vi "Watts Up Series Real Time Graph.vi"() -> ()   [LabVIEW 2013]
doc: "Graph data from the Watts Up in a live-stream type format. This requires the use of <b>External logging mode</b> for the Watts Up device. The data will not be saved on the Watts Up meter but rather into the chart itself. To retrieve the data from the chart, right click and use <b>Export</b>.\n\nWhen <b>STOP</b> is pressed, the meter will be set back into internal logging mode (however the data will be cleared anytime the logging mode is changed)."
uses:
  <instrlib>/Watts Up Series/Watts Up Series.lvlib
panel:
  in  "Relay (ON)":bool=TRUE
  in  "Items To Graph":bool[](array[boolean])=[FALSE, FALSE, FALSE, FALSE, FALSE, FALSE, FALSE, FALSE, FALSE, FALSE, FALSE, FALSE, FALSE, FALSE, FALSE, FALSE, FALSE, FALSE]
  in  "Interval (10 s)":i32=10
  in  "?":bool
  out "Waveform Chart":T1(graph)
  in  "VISA resource name":refnum<visa-resource-name>
  # "(c) 2014 NATIONAL INSTRUMENTS.  ALL RIGHTS RESERVED."
  # "Watts"
  # "Volts"
  # "Amps"
  # "Watt Hours"
  # "Cost"
  # "WH/Month"
  # "Cost/Month"
  # "Wmax"
  # "Vmax"
  # "Amax"
  # "Wmin"
  # "Vmin"
  # "Amin"
  # "Power Factor"
  # "Duty Cycle"
  # "Power Cycle"
  # "Line Freq."
  # "Volt-Amps"
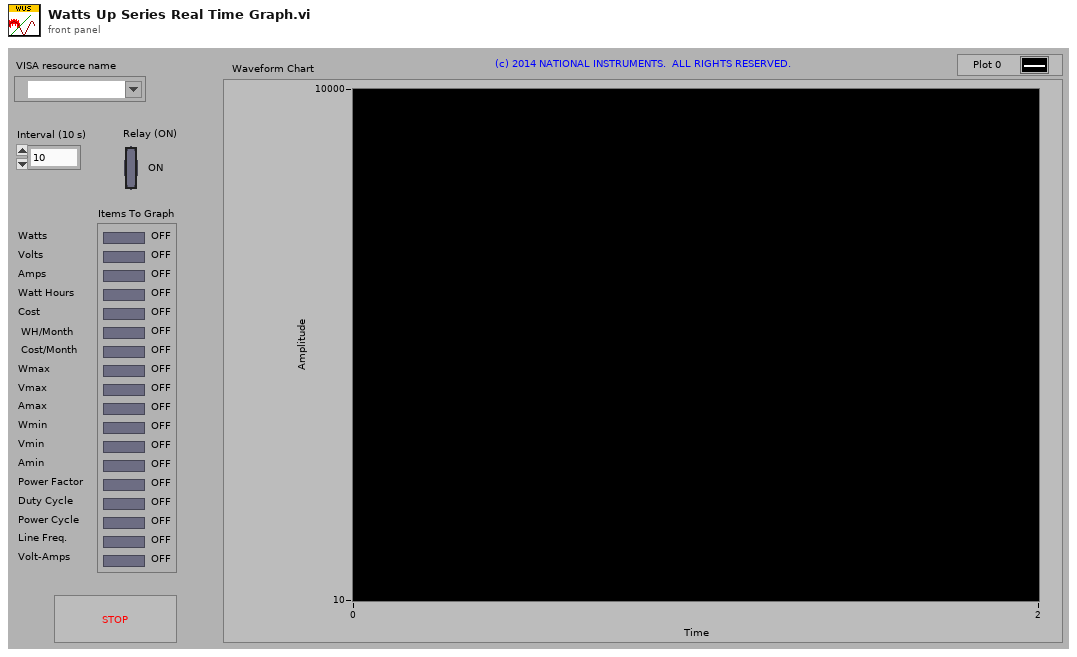
[diagram p1: front panel]
types:
  T1 = cluster{"Record[0]":dbl, "Record[1]":dbl, "Record[2]":dbl, "Record[3]":dbl, "Record[4]":dbl, "Record[5]":dbl, "Record[6]":dbl, "Record[7]":dbl, "Record[8]":dbl}
  T2 = cluster{"[0]":dbl, "[1]":dbl, "[2]":dbl, "[3]":dbl, "[4]":dbl, "[5]":dbl, "[6]":dbl, "[7]":dbl, "[8]":dbl}
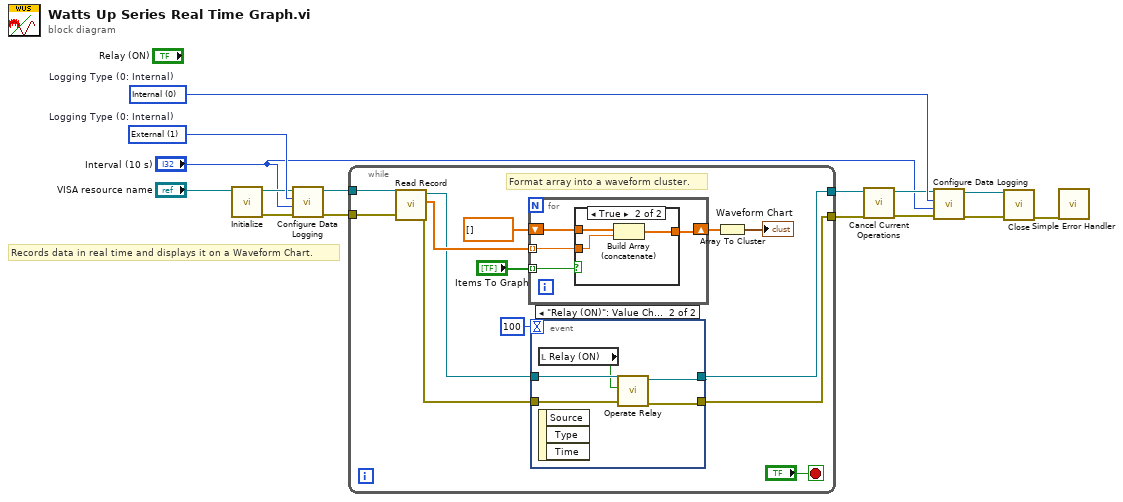
[diagram p0: block diagram]
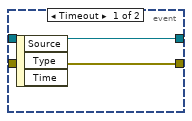
[diagram p2: hidden frame]
diagram:
  w10 = 0 items=["Internal", "External", "TCP"]  # Logging Type (0: Internal)
  w14 = 1 items=["Internal", "External", "TCP"]  # Logging Type (0: Internal)
  # "Records data in real time and displays it on a Waveform Chart."
  n1 = call <instrlib>:"Initialize.vi"("VISA resource name"="VISA resource name") -> ("error out"=w11:errorcluster, "VISA resource name out"=w12:refnum<visa-resource-name>)  [unwired: 9 in]
  n2 = call <instrlib>:"Configure Data Logging.vi"("error in (no error)"=w11, "Interval (10 s)"="Interval (10 s)", "Logging Type (0: Internal)"=w14, "VISA resource name"=w12) -> ("error out"=w2:errorcluster, "VISA resource name out"=w1:refnum<visa-resource-name>)  [unwired: 6 in]
  n3 = while {
    tunnel: w1 -> [w27]
    tunnel: w2 -> [w26]
    tunnel: [w18] -> w4
    tunnel: [w17] -> w3
    stop <- "?" stop-if-true
    # "Format array into a waveform cluster."
    n4 = call <instrlib>:"Read Record.vi"("error in (no error)"=w26, "VISA resource name"=w27) -> ("error out"=w20:errorcluster, "Record"=w25:dbl[], "VISA resource name out"=w19:refnum<visa-resource-name>)  [unwired: 7 in]
    n5 = for {
      shift-right: [w36] -> w21
      shift-left: dbl[] [] -> [w39]
      tunnel: w25 -> [w38] mode=indexing
      tunnel: "Items To Graph" -> [w37] mode=indexing
      n6 = case shown="True" w37 {
        tunnel: w39 -> [w40 w43]
        tunnel: w38 -> [_ w42]
        tunnel: [w40 w41] -> w36
        frame False {
        }
        frame True {
          n7 = Build Array (concatenate)(w43, w42) -> (w41:dbl[])
        }
      }
    }
    n8 = event shown="[1] \"Relay (ON)\": Value Change" {
      selector: _ -> [_ _]
      dyn-events: _ -> [_ _]
      timeout: 100 -> [_ _]
      tunnel: w20 -> [w29 w34]
      tunnel: w19 -> [w30 w35]
      tunnel: [w30 w32] -> w18
      tunnel: [w29 w31] -> w17
      event Timeout {
        n9 = event-data() -> ()  [unwired: 1 in, 3 out]
      }
      event "Relay (ON)": Value Change {
        n10 = local read "Relay (ON)"() -> (w33:bool)
        n11 = event-data() -> ()  [unwired: 1 in, 3 out]
        n12 = call <instrlib>:"Operate Relay.vi"("error in (no error)"=w34, "Relay (ON)"=w33, "VISA resource name"=w35) -> ("error out"=w31:errorcluster, "VISA resource name out"=w32:refnum<visa-resource-name>)  [unwired: 7 in]
      }
    }
    n13 = Array To Cluster(array=w21) -> (cluster=→"Waveform Chart":T2)
  }
  n14 = call <instrlib>:"Cancel Current Operations.vi"("error in (no error)"=w3, "VISA resource name"=w4) -> ("error out"=w6:errorcluster, "VISA resource name out"=w7:refnum<visa-resource-name>)  [unwired: 8 in]
  n15 = call <instrlib>:"Configure Data Logging.vi"("error in (no error)"=w6, "Interval (10 s)"="Interval (10 s)", "Logging Type (0: Internal)"=w10, "VISA resource name"=w7) -> ("error out"=w8:errorcluster, "VISA resource name out"=w9:refnum<visa-resource-name>)  [unwired: 6 in]
  n16 = call <instrlib>:"Close.vi"("error in (no error)"=w8, "VISA resource name"=w9) -> ("error out"=w13:errorcluster)  [unwired: 9 in]
  n17 = call <vilib>:"Simple Error Handler.vi"("error in (no error)"=w13) -> ()  [unwired: 4 in, 5 out]
